vi "Text_File_Driver.vi"(0 "Data_In":string, 1 "Config_File_Path":path, 11 "Error_Out":errorcluster, 13 "INI_Operation_Select":T1=enum."Write") -> (4 "Data_Out":string, 15 "Error_Out":errorcluster)   [LabVIEW 2021]
doc: "Used to read and write the Text file"
uses:
  Controls/Text_File_Operation_Select.ctl
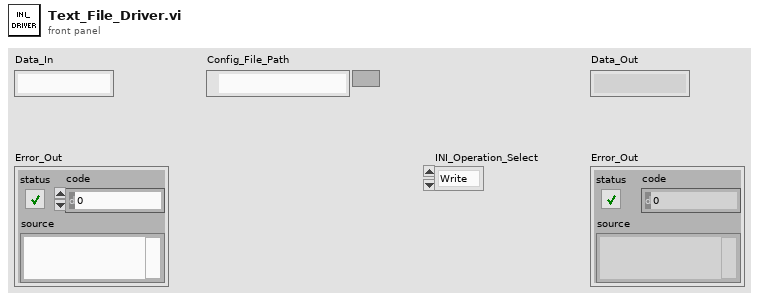
[diagram p1: front panel]
types:
  T1 = typedef "Text_File_Operation_Select.ctl" = enum16{"Initialize", "Read", "Write"}
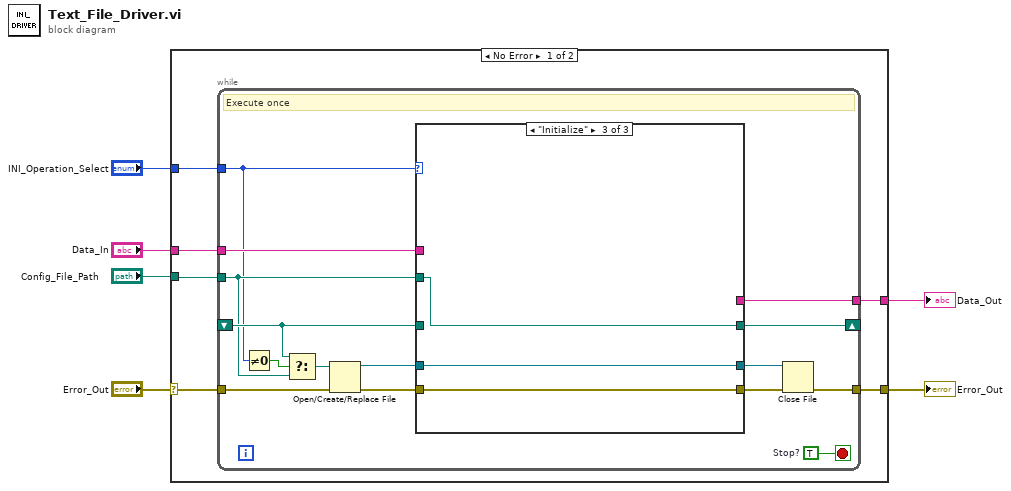
[diagram p0: block diagram]
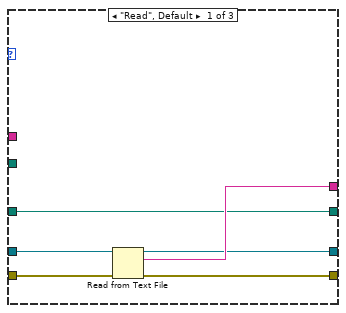
[diagram p2: hidden frame]
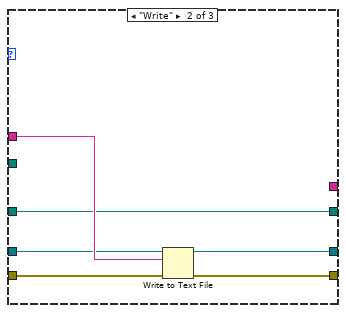
[diagram p3: hidden frame]
diagram:
  n1 = case shown="No Error" "Error_Out" {
    selector: "Error_Out" -> [w10 w43]
    tunnel: "INI_Operation_Select" -> [w12 _]
    tunnel: [w11 w43] -> w4
    tunnel: "Data_In" -> [w9 _]
    tunnel: "Config_File_Path" -> [w8 _]
    tunnel: [w7 _] -> w1
    frame No Error {
      n2 = while {
        tunnel: w12 -> [w13]
        tunnel: [w19] -> w11
        tunnel: w10 -> [w26]
        tunnel: w9 -> [w24]
        shift-right: [w22] -> _
        shift-left: _ -> [w16]
        tunnel: w8 -> [w15]
        tunnel: [w23] -> w7
        stop <- w27 stop-if-true
        w27 = TRUE  # Stop?
        # "Execute once"
        n3 = Not Equal To 0?(x=w13) -> (x != 0?=w14:bool)
        n4 = Select(t=w16, s=w14, f=w15) -> (s? t:f=w17:path)
        n5 = Open/Create/Replace File(file path (use dialog)=w17, error in=w26) -> (refnum out=w20:refnum<file>, error out=w21:errorcluster)  [unwired: 4 in, 1 out]
        n6 = case shown="\"Initialize\"" w13 {
          tunnel: [w32 w39 w41] -> w25
          tunnel: w21 -> [w33 w37 w41]
          tunnel: w15 -> [_ _ w42]
          tunnel: w20 -> [w31 w35 w40]
          tunnel: w24 -> [_ w38 _]
          tunnel: [w30 _ _] -> w23
          tunnel: [w28 w36 w42] -> w22
          tunnel: w16 -> [w28 w36 _]
          tunnel: [w29 w34 w40] -> w18
          frame "Read", Default {
            n7 = Read from Text File(file (use dialog)=w31, error in=w33) -> (refnum out=w29:refnum<file>, text=w30:string, error out=w32:errorcluster)  [unwired: 2 in, 1 out]
          }
          frame "Write" {
            n8 = Write to Text File(file (use dialog)=w35, text=w38, error in=w37) -> (refnum out=w34:refnum<file>, error out=w39:errorcluster)  [unwired: 1 in, 1 out]
          }
          frame "Initialize" {
          }
        }
        n9 = Close File(refnum=w18, error in=w25) -> (error out=w19:errorcluster)  [unwired: 1 out]
      }
    }
    frame Error {
    }
  }
  "Error_Out" <- w4
  "Data_Out" <- w1
